vi "updateCurrentScore.vi"(8 "error in (no error)":errorcluster, 11 "Player in":refnum<class "Player.lvclass">) -> (0 "error out":errorcluster, 3 "Player out":refnum<class "Player.lvclass">)   [LabVIEW 2019, in "Player.lvclass"]
uses:
  Player.lvclass
  Player.lvclass/Player.ctl
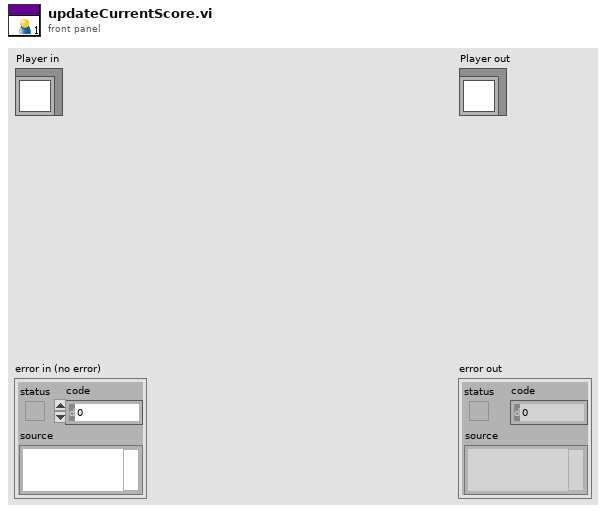
[diagram p1: front panel]
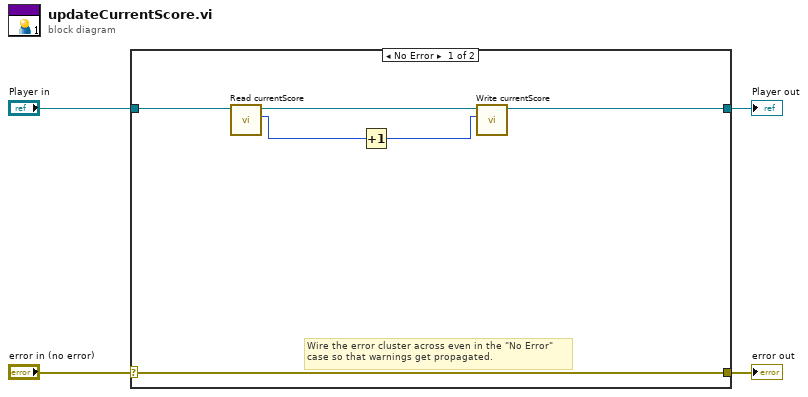
[diagram p0: block diagram]
diagram:
  n1 = case shown="No Error" "error in (no error)" {
    selector: "error in (no error)" -> [w9 w12]
    tunnel: [w9 w12] -> w3
    tunnel: [w6 w11] -> w1
    tunnel: "Player in" -> [w10 w11]
    frame No Error {
      # "Wire the error cluster across even in the \"No Error\"\ncase so that warnings get propagated."
      n2 = call "Read currentScore.vi"("Player in"=w10) -> ("currentScore"=w7:u64, "Player out"=w8:refnum<class "Player.lvclass">)  [unwired: 8 in, 1 out]
      n3 = Increment(x=w7) -> (x+1=w5:u64)
      n4 = call "Write currentScore.vi"("currentScore"=w5, "Player in"=w8) -> ("Player out"=w6:refnum<class "Player.lvclass">)  [unwired: 8 in, 1 out]
    }
    frame Error {
    }
  }
  "error out" <- w3
  "Player out" <- w1
